vi "Heading.vi"(4 "Class (\"\")":string, 5 "Level (1)":u8=1 min=1 max=6 step=1, 6 "Heading (\"\")":string, 7 "Previous HTML in":string) -> (3 "HTML out":string)   [LabVIEW 2011]
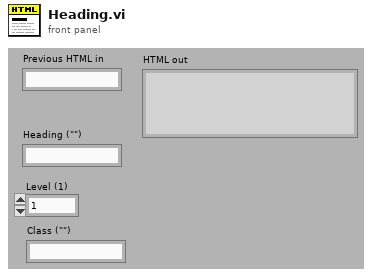
[diagram p1: front panel]
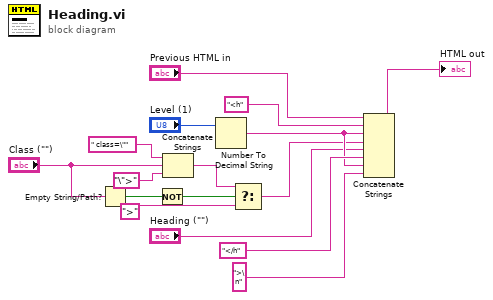
[diagram p0: block diagram]
diagram:
  n1 = Empty String/Path?(string/path="Class (\"\")") -> (empty?=w10:bool)
  n2 = Not(x=w10) -> (.not. x?=w6:bool)
  n3 = Concatenate Strings(" class=\"", "Class (\"\")", "\">") -> (w8:string)
  n4 = Number To Decimal String(number="Level (1)") -> (decimal integer string=w12:string)  [unwired: 1 out]
  n5 = Select(t=w8, s=w6, f=">") -> (s? t:f=w4:string)
  n6 = Concatenate Strings("Previous HTML in", "<h", w12, w4, "Heading (\"\")", "</h", w12, ">\n") -> (→"HTML out":string)
